vi "python analysis.vi"(6 "function name":string, 7 "Numeric":dbl, 9 "Waveforms":waveform(dbl)[](array[waveform]), 10 "module path":path, 11 "Refnum in":refnum<k35>) -> (3 "dt":dbl)   [LabVIEW 2020, in "picoscope.lvclass"]
uses:
  picoscope.lvclass
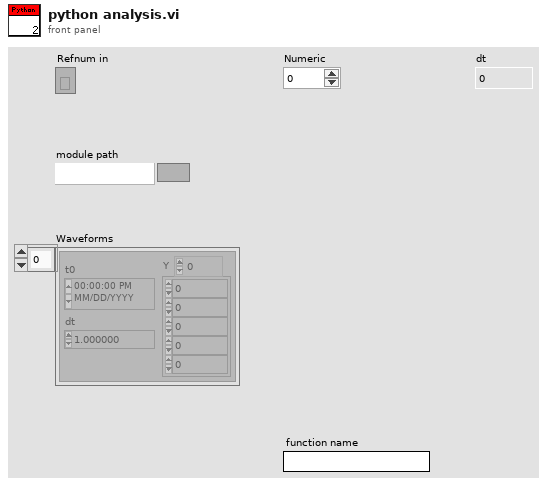
[diagram p1: front panel]
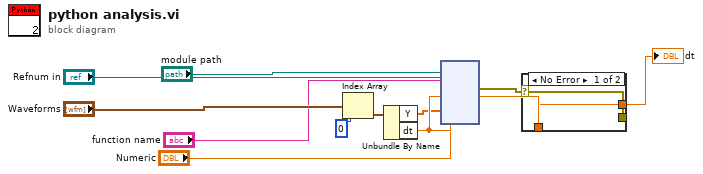
[diagram p0: block diagram]
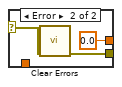
[diagram p2: hidden frame]
diagram:
  n1 = Index Array(array="Waveforms", index=0 ("disabled index (col)")) -> (element=w5:waveform(dbl))
  n2 = Unbundle By Name(w5) -> ("Y"=w7:dbl[], "dt"=w9:dbl)
  n3 = node("Refnum in", "module path", "function name", w9, w7, w9, "Numeric") -> (w10:errorcluster, w11:dbl)  [unwired: 4 in, 3 out]
  n4 = case shown="No Error" w10 {
    selector: w10 -> [w13 w16]
    tunnel: w11 -> [w14 _]
    tunnel: [w14 0.0 ("dt")] -> w12
    tunnel: [w13 w15] -> _
    frame No Error {
    }
    frame Error {
      n5 = call <vilib>:"Clear Errors.vi"("error in (no error)"=w16) -> ("error out"=w15:errorcluster)  [unwired: 5 in, 1 out]
    }
  }
  "dt" <- w12
